vi "Progress_Set Target.vi"(8 "error in (no error)":errorcluster, 10 "Set Target":i32, 11 "Dependency Source in":refnum<class "Dependency Source.lvclass">) -> (0 "error out":errorcluster, 3 "Dependency Source out":refnum<class "Dependency Source.lvclass">)   [LabVIEW 2019, in "Project.Dependencies Finder.lvlib" / "Dependency Source.lvclass"]
uses:
  Dependency Source.lvclass
  Dependency Source.lvclass/Dependency Source.ctl
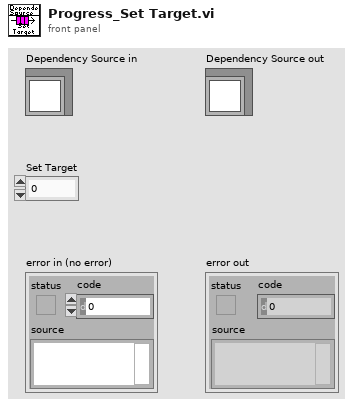
[diagram p1: front panel]
types:
  T1 = typedef "Project.Dependencies Finder.lvlib/Ctl_Progress Queue.ctl" = refnum<queue>
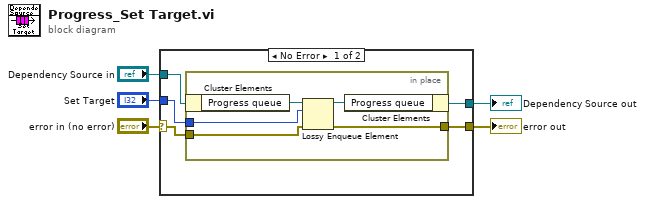
[diagram p0: block diagram]
diagram:
  n1 = case shown="No Error" "error in (no error)" {
    selector: "error in (no error)" -> [w8 w17]
    tunnel: [w7 w17] -> w4
    tunnel: [w10 w16] -> w2
    tunnel: "Dependency Source in" -> [w9 w16]
    tunnel: "Set Target" -> [w6 _]
    frame No Error {
      n2 = in-place {
        in-place-border: w8 -> [w12]
        in-place-border: [w13] -> w7
        in-place-border: w6 -> [w11]
        n3 = in-place-cluster #1(w9) -> ("Progress queue"=w15:T1)
        n4 = Lossy Enqueue Element(queue=w15, element=w11, error in (no error)=w12) -> (queue out=w14:T1, error out=w13:errorcluster)  [unwired: 2 out]
        n5 = in-place-cluster #1("Progress queue"=w14) -> (w10:refnum<class "Dependency Source.lvclass">)
      }
    }
    frame Error {
    }
  }
  "error out" <- w4
  "Dependency Source out" <- w2
